vi "Constructor by Table.vi"(8 "error in (no error)":errorcluster, 10 "Configured Table":refnum<class "Basic Table.lvclass">, 11 "Form from Configured Table in":refnum<class "Form from Configured Table.lvclass">) -> (0 "error out":errorcluster, 3 "Form from Configured Table out":refnum<class "Form from Configured Table.lvclass">)   [LabVIEW 2020, in "Panel Form Controller.lvlib" / "Form from Configured Table.lvclass"]
uses:
  Form from Configured Table.lvclass
  Database OOP/Table Libraries/Basic Table/Basic Table Class/Basic Table.lvclass
  Form from Configured Table.lvclass/Form from Configured Table.ctl
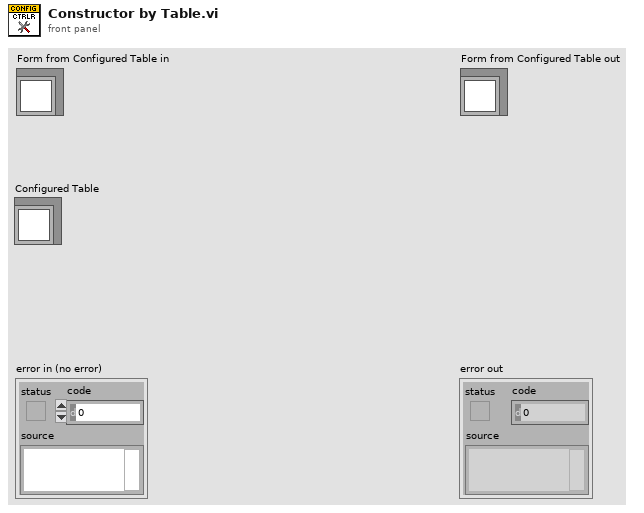
[diagram p1: front panel]
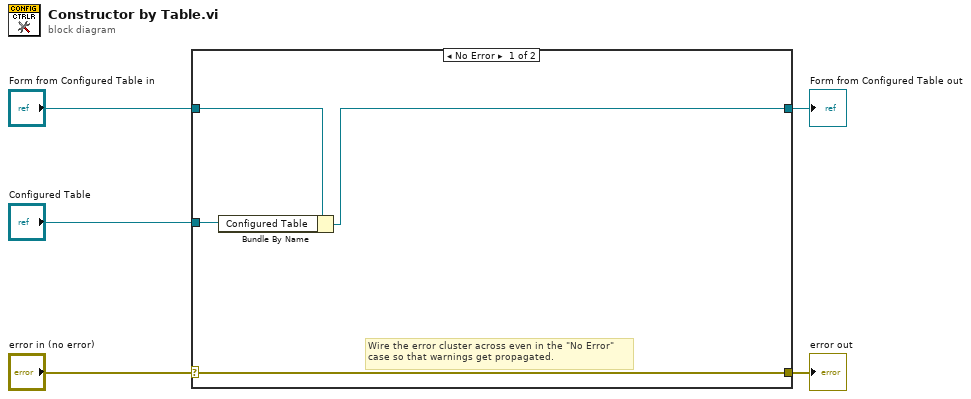
[diagram p0: block diagram]
diagram:
  n1 = case shown="No Error" "error in (no error)" {
    selector: "error in (no error)" -> [w9 w11]
    tunnel: [w9 w11] -> w4
    tunnel: [w6 w10] -> w2
    tunnel: "Form from Configured Table in" -> [w8 w10]
    tunnel: "Configured Table" -> [w7 _]
    frame No Error {
      # "Wire the error cluster across even in the \"No Error\"\ncase so that warnings get propagated."
      n2 = Bundle By Name(cluster=w8, "Configured Table"=w7) -> (w6:refnum<class "Form from Configured Table.lvclass">)
    }
    frame Error {
    }
  }
  "error out" <- w4
  "Form from Configured Table out" <- w2
